vi "Report Execution Error.vi"(8 "error in (no error)":errorcluster) -> ()   [LabVIEW 2020, in "FlexBlocks.lvlib"]
uses:
  FlexBlocks.lvlib
  <vilib>/Utility/miscctls.llb/LVMapReplaceAction.ctl
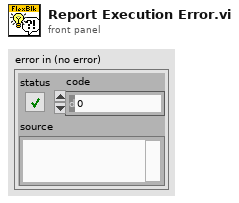
[diagram p1: front panel]
types:
  T1 = typedef "LVMapReplaceAction.ctl" = enum32{"Modify Entry only if found", "Add or Modify Entry", "Delete Entry"}
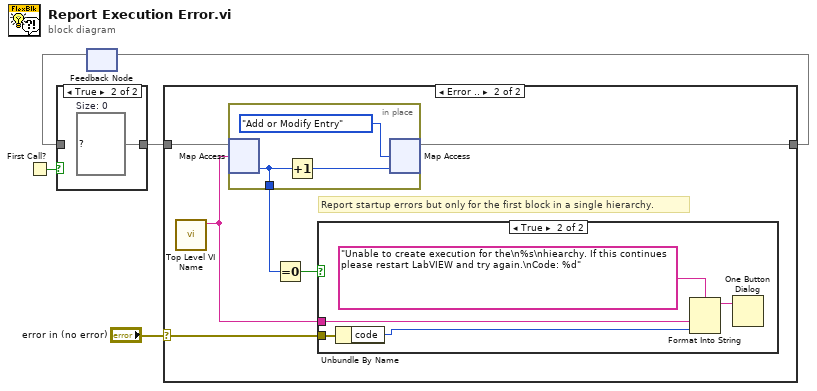
[diagram p0: block diagram]
diagram:
  n1 = First Call?() -> (First Call?: T/F=w5:bool)
  n2 = feedback #1() -> (w4:map{string, i32})  [unwired: 1 in]
  n3 = case shown="True" w5 {
    tunnel: [w6 w7] -> w2
    tunnel: w4 -> [w6 _]
    frame False {
    }
    frame True {
      w7 = map{string, i32} {}  # Size: 0
    }
  }
  n4 = case shown="Error .." "error in (no error)" {
    selector: "error in (no error)" -> [_ w13]
    tunnel: w2 -> [w8 w12]
    tunnel: [w8 w9] -> w1
    frame No Error {
    }
    frame Error {
      # "Report startup errors but only for the first block in a single hierarchy."
      n5 = call "Top Level VI Name.vi"() -> ("Top Level VI Name"=w11:string)  [unwired: 11 in]
      n6 = in-place {
        in-place-border: [w17] -> w10
        n7 = in-place-map #2(w12, w11) -> (w17:i32)  [unwired: 1 in, 1 out]
        n8 = Increment(x=w17) -> (x+1=w16:i32)
        n9 = in-place-map #2(w16, LVMapReplaceAction."Add or Modify Entry" ("action")) -> (w9:map{string, i32})  [unwired: 2 out]
      }
      n10 = Equal To 0?(x=w10) -> (x = 0?=w14:bool)
      n11 = case shown="True" w14 {
        tunnel: w11 -> [_ w21]
        tunnel: w13 -> [_ w19]
        frame False {
        }
        frame True {
          n12 = Unbundle By Name(w19) -> ("code"=w18:i32)
          n13 = Format Into String(format string="Unable to create execution for the\n%s\nhiearchy. If this continues please restart LabVIEW and try again.\nCode: %d", w21, w18) -> (resulting string=w20:string)  [unwired: 2 in, 1 out]
          n14 = One Button Dialog(message=w20) -> ()  [unwired: 1 in, 1 out]
        }
      }
    }
  }
  n15 = feedback-in #1(w1) -> ()
